vi "UpdateUI.vi"(8 "error in (no error)":errorcluster, 9 "Json Data":string, 10 "Type":string, 11 "VisionUI in":refnum<class "VisionUI.lvclass">) -> (0 "error out":errorcluster, 3 "VisionUI out":refnum<class "VisionUI.lvclass">)   [LabVIEW 2019, in "VisionUI.lvlib" / "VisionUI.lvclass"]
uses:
  VisionUI.lvclass
  VisionUI.lvclass/VisionUI.ctl
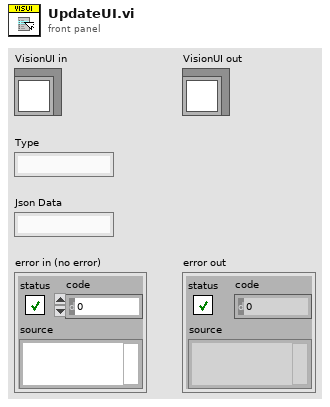
[diagram p1: front panel]
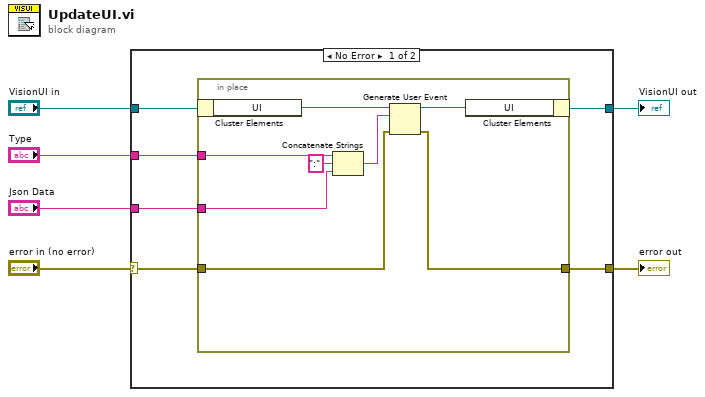
[diagram p0: block diagram]
diagram:
  n1 = case shown="No Error" "error in (no error)" {
    selector: "error in (no error)" -> [w9 w22]
    tunnel: [w8 w22] -> w5
    tunnel: [w7 w21] -> w3
    tunnel: "VisionUI in" -> [w12 w21]
    tunnel: "Type" -> [w11 _]
    tunnel: "Json Data" -> [w10 _]
    frame No Error {
      n2 = in-place {
        in-place-border: w11 -> [w18]
        in-place-border: w10 -> [w16]
        in-place-border: w9 -> [w14]
        in-place-border: [w13] -> w8
        n3 = in-place-cluster #1(w12) -> ("UI"=w20:refnum<user-event>)
        n4 = Concatenate Strings(w18, ":" ("string"), w16) -> (w15:string)
        n5 = Generate User Event(user event=w20, event data cluster=w15, error in=w14) -> (user event out=w19:refnum<user-event>, error out=w13:errorcluster)  [unwired: 1 in]
        n6 = in-place-cluster #1("UI"=w19) -> (w7:refnum<class "VisionUI.lvclass">)
      }
    }
    frame Error {
    }
  }
  "error out" <- w5
  "VisionUI out" <- w3
